vi "Set Initialization Data - TCP Listener.vi"(8 "error in":errorcluster, 11 "TCP Server in":refnum<class "TCP Server.lvclass">) -> (0 "error out":errorcluster, 3 "TCP Server out":refnum<class "TCP Server.lvclass">)   [LabVIEW 2017, in "TCP Server.lvlib" / "TCP Server.lvclass"]
doc: "In this VI you can set the initialization data of a statically-linked subWorker."
uses:
  TCP Server.lvclass
  TCP Listener/Initialization Data.ctl
  TCP Listener/Response Cases.ctl
  <vilib>/addons/_Workers/Library/Case Label.ctl
  TCP Server.lvclass/TCP Server.ctl
  TCP Listener/TCP Listener.lvclass
  C:/Program Files (x86)/National Instruments/LabVIEW 2017/vi.lib/addons/_Workers/Library/Classes/Worker/Worker.lvclass
  <vilib>/addons/_Workers/Library/Workers.lvlib
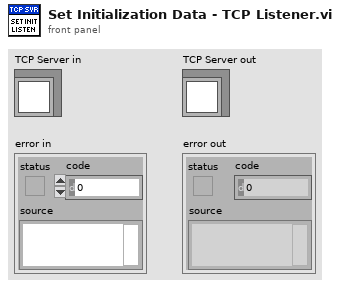
[diagram p1: front panel]
types:
  T1 = typedef "TCP Server.lvlib/TCP Listener.lvclass/Initialization Data.ctl" = cluster{"Response Cases":T2}
  T2 = typedef "TCP Server.lvlib/TCP Listener.lvclass/Response Cases.ctl" = cluster{"Add Listener":T3, "New Connection":T3}
  T3 = typedef "Workers.lvlib/Case Label.ctl" = string
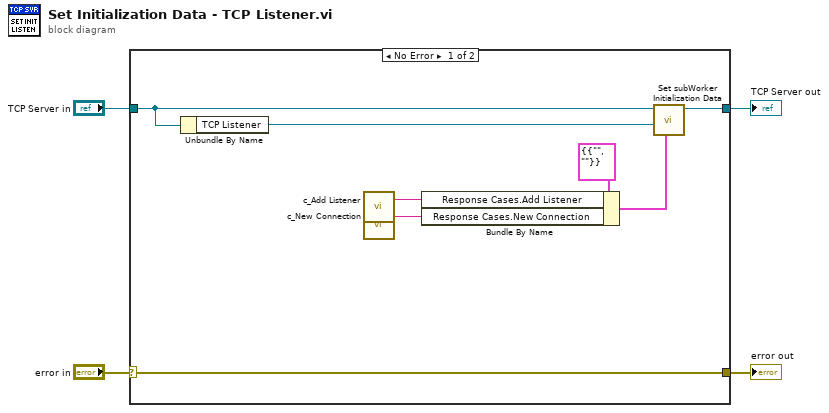
[diagram p0: block diagram]
diagram:
  n1 = case shown="No Error" "error in" {
    selector: "error in" -> [w12 w14]
    tunnel: [w12 w14] -> w3
    tunnel: [w10 w13] -> w2
    tunnel: "TCP Server in" -> [w9 w13]
    frame No Error {
      n2 = Unbundle By Name(w9) -> ("TCP Listener"=w11:refnum<class "TCP Listener.lvclass">)
      n3 = call "c_Add Listener.vi"() -> ("Case Label"=w6:T3)  [unwired: 1 in]
      n4 = call "c_New Connection.vi"() -> ("Case Label"=w5:T3)  [unwired: 1 in]
      n5 = Bundle By Name(cluster=T1 {"Response Cases"={"Add Listener"="", "New Connection"=""}} ("Initialization Data"), "Response Cases.Add Listener"=w6, "Response Cases.New Connection"=w5) -> (w7:T1)
      n6 = call-dynamic "Set subWorker Initialization Data.vi"("Initialization Data"=w7, "subWorker"=w11, "Worker"=w9) -> ("Worker out"=w10:refnum<class "TCP Server.lvclass">)  [unwired: 8 in]
    }
    frame Error {
    }
  }
  "error out" <- w3
  "TCP Server out" <- w2
